vi "WaveformName.vi"(11 "signal in":waveform(sgl)) -> (2 "name":string, 3 "signal out":waveform(sgl))   [LabVIEW 2017]
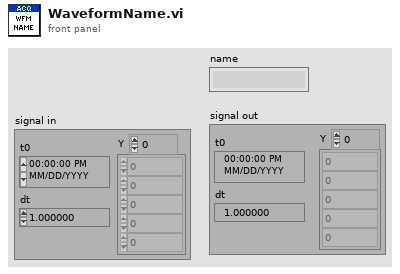
[diagram p1: front panel]
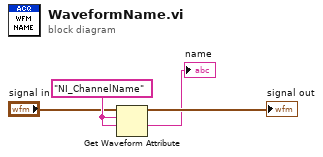
[diagram p0: block diagram]
diagram:
  w2 = "NI_ChannelName" ("name")
  n1 = Get Waveform Attribute(5:w2, 6:w2, 7:"signal in") -> (1:→"name":string, 3:→"signal out":waveform(sgl))  [unwired: 1 in, 2 out]
